vi "Show Battery Voltage.vi"(8 "error in (no error)":errorcluster) -> (0 "error out":errorcluster)   [LabVIEW 2015]
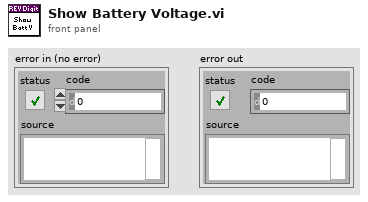
[diagram p1: front panel]
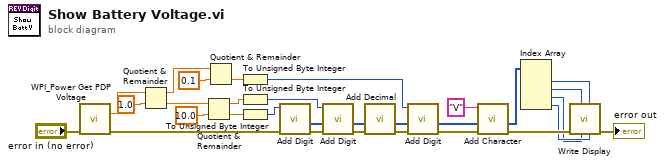
[diagram p0: block diagram]
diagram:
  n1 = call <vilib>:"WPI_Power Get PDP Voltage.vi"("error in"="error in (no error)") -> ("voltage (V)"=w2:dbl, "error out"=w19:errorcluster)  [unwired: 13 in]
  n2 = Quotient & Remainder(x=w2, y=1.0) -> (x-y*floor(x/y)=w4:dbl, floor(x/y)=w6:dbl)
  n3 = Quotient & Remainder(x=w6, y=10.0) -> (x-y*floor(x/y)=w21:dbl, floor(x/y)=w20:dbl)
  n4 = Quotient & Remainder(x=w4, y=0.1) -> (floor(x/y)=w22:dbl)  [unwired: 1 out]
  n5 = To Unsigned Byte Integer(number=w22) -> (unsigned 8bit integer=w30:u8)
  n6 = To Unsigned Byte Integer(number=w21) -> (unsigned 8bit integer=w29:u8)
  n7 = To Unsigned Byte Integer(number=w20) -> (unsigned 8bit integer=w28:u8)
  n8 = call "Add Digit.vi"("error in (no error)"=w19, "Digit"=w28) -> ("error out"=w8:errorcluster, "Output Array"=w9:u16[])  [unwired: 8 in]
  n9 = call "Add Digit.vi"("error in (no error)"=w8, "Input Array"=w9, "Digit"=w29) -> ("error out"=w11:errorcluster, "Output Array"=w10:u16[])  [unwired: 7 in]
  n10 = call "Add Decimal.vi"("error in (no error)"=w11, "Input Array"=w10) -> ("error out"=w12:errorcluster, "Output Array"=w13:u16[])  [unwired: 8 in]
  n11 = call "Add Digit.vi"("error in (no error)"=w12, "Input Array"=w13, "Digit"=w30) -> ("error out"=w23:errorcluster, "Output Array"=w24:u16[])  [unwired: 7 in]
  n12 = call "Add Character.vi"("error in (no error)"=w23, "Input Array"=w24, "Character"="V") -> ("error out"=w26:errorcluster, "Output Array"=w25:u16[])  [unwired: 7 in]
  n13 = Index Array(array=w25) -> (element #1=w14:u16, element #2=w15:u16, element #3=w16:u16, element #4=w17:u16)  [unwired: 4 in]
  n14 = call "Write Display.vi"("D3"=w17, "D0"=w14, "D2"=w16, "D1"=w15, "error in (no error)"=w26) -> ("error out"=→"error out":errorcluster)  [unwired: 6 in]
